vi "FCI Arrow Points.vi"(0 "Max Edge Points":cluster{"X":sgl, "Y":sgl}[](array[cluster]) {"Y" format="%.2f"; "X" format="%.2f"}, 5 "Search Lines":T3[](array[typedef]) {"Edge Info"."Distance (Real-World)" format="%.2f"; "Edge Info"."Location (Real-World)"."Y" format="%.2g"; "Edge Info"."Location (Real-World)"."X" format="%.2f"; "Edge Info"."Noise" format="%.2f"; "Edge Info"."Location (Pixel)"."Y" format="%.2g"; "Edge Info"."Location (Pixel)"."X" format="%.2f"; "Edge Info"."Strength" format="%.2f"; "Edge Info"."Distance (Pixel)" format="%.2f"}, 7 "Edge Last Points":cluster{"X":sgl, "Y":sgl}[](array[cluster]), 9 "Edge First Points":cluster{"X":sgl, "Y":sgl}[](array[cluster]), 11 "error constant":errorcluster) -> (6 "First Arrow Line Coord":T1, 8 "Second Arrow Line Coord":T2, 13 "Max first Arrow Line Coord out":T1, 14 "Max Last Arrow Line Coord out":T1, 15 "error IO":errorcluster)   [LabVIEW 2019, in "Algorithm.lvclass"]
uses:
  FrameworkOverrides/Algorithm.lvclass
  <vilib>/vision/Measure.llb/Edge New.ctl
  <vilib>/vision/Measure.llb/Search Line.ctl
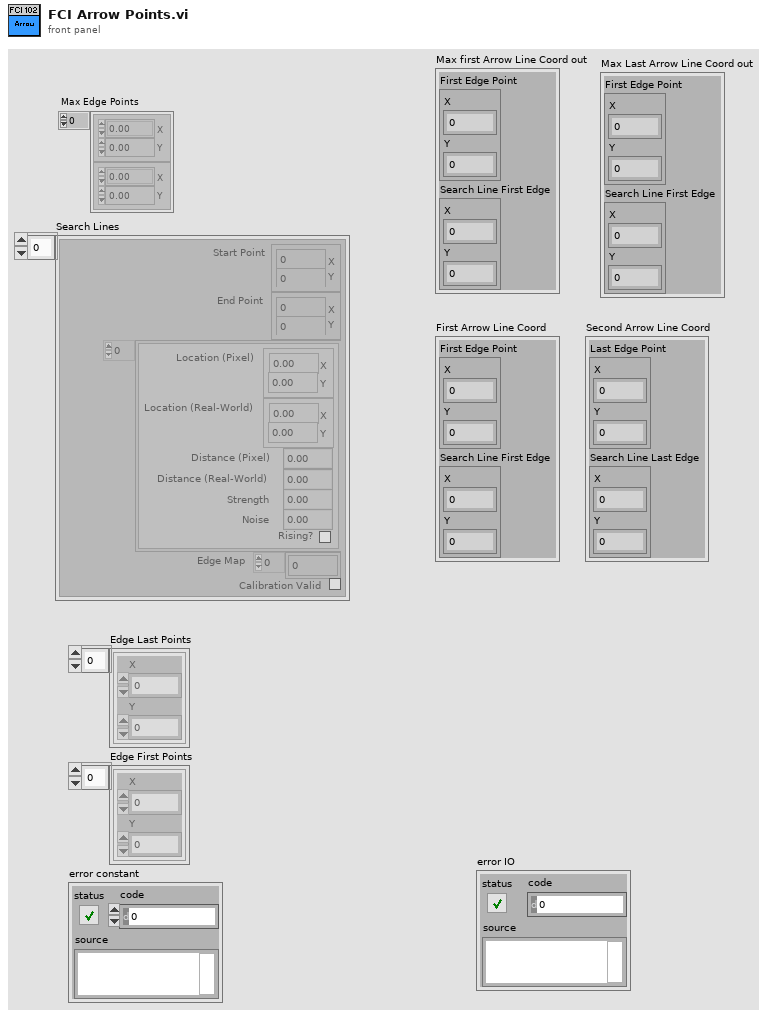
[diagram p1: front panel]
types:
  T1 = cluster{"First Edge Point":cluster{"X":sgl, "Y":sgl}, "Search Line First Edge":cluster{"X":sgl, "Y":sgl}}
  T2 = cluster{"Last Edge Point":cluster{"X":sgl, "Y":sgl}, "Search Line Last Edge":cluster{"X":sgl, "Y":sgl}}
  T3 = typedef "Search Line.ctl" = cluster{"Start Point":cluster{"X":sgl, "Y":sgl}, "End Point":cluster{"X":sgl, "Y":sgl}, "Edge Info":T4[], "Edge Map":dbl[], "Calibration Valid":bool}
  T4 = typedef "Edge New.ctl" = cluster{"Location (Pixel)":cluster{"X":sgl, "Y":sgl}, "Location (Real-World)":cluster{"X":sgl, "Y":sgl}, "Distance (Pixel)":dbl, "Distance (Real-World)":dbl, "Strength":dbl, "Noise":dbl, "Rising?":bool}
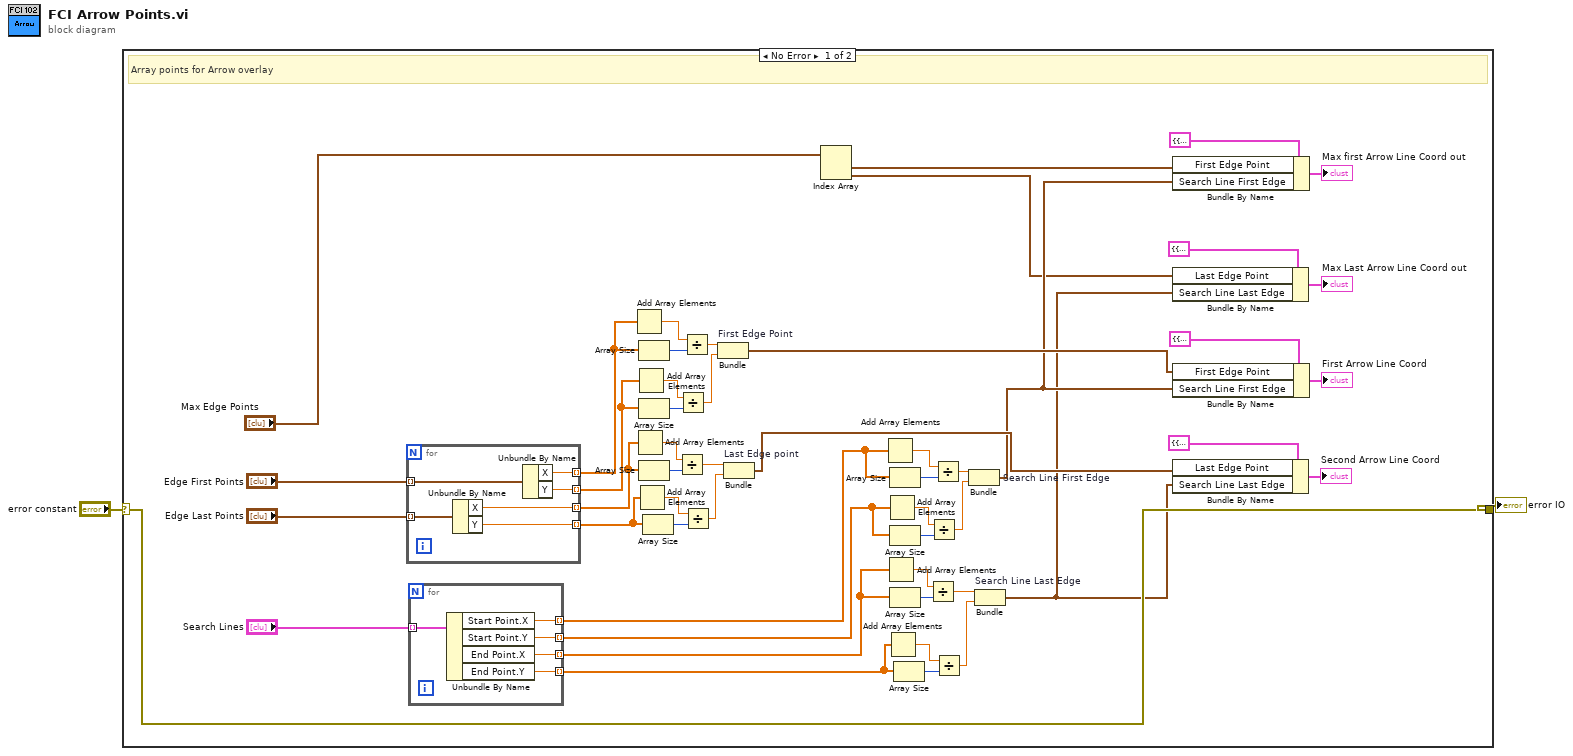
[diagram p0: block diagram]
diagram:
  n1 = case shown="No Error" "error constant" {
    selector: "error constant" -> [w18 w65]
    tunnel: [w18 w65] -> w1
    frame No Error {
      # "Array points for Arrow overlay"
      n2 = for {
        tunnel: "Edge Last Points" -> [w63] mode=indexing
        tunnel: "Edge First Points" -> [w64] mode=indexing
        tunnel: [w62] -> w37 mode=indexing
        tunnel: [w61] -> w41 mode=indexing
        tunnel: [w60] -> w46 mode=indexing
        tunnel: [w59] -> w50 mode=indexing
        n3 = Unbundle By Name(w63) -> ("X"=w60:sgl, "Y"=w59:sgl)
        n4 = Unbundle By Name(w64) -> ("X"=w62:sgl, "Y"=w61:sgl)
      }
      n5 = for {
        tunnel: "Search Lines" -> [w58] mode=indexing
        tunnel: [w57] -> w22 mode=indexing
        tunnel: [w56] -> w21 mode=indexing
        tunnel: [w55] -> w20 mode=indexing
        tunnel: [w54] -> w19 mode=indexing
        n6 = Unbundle By Name(w58) -> ("Start Point.X"=w57:sgl, "Start Point.Y"=w56:sgl, "End Point.X"=w55:sgl, "End Point.Y"=w54:sgl)
      }
      n7 = Add Array Elements(numeric array=w37) -> (sum=w36:sgl)
      n8 = Add Array Elements(numeric array=w46) -> (sum=w44:sgl)
      n9 = Add Array Elements(numeric array=w41) -> (sum=w40:sgl)
      n10 = Add Array Elements(numeric array=w50) -> (sum=w48:sgl)
      n11 = Array Size(array=w37) -> (size(s)=w38:i32)
      n12 = Array Size(array=w41) -> (size(s)=w42:i32)
      n13 = Array Size(array=w46) -> (size(s)=w45:i32)
      n14 = Array Size(array=w50) -> (size(s)=w49:i32)
      n15 = Divide(x=w44, y=w45) -> (x/y=w43:sgl)
      n16 = Divide(x=w40, y=w42) -> (x/y=w39:sgl)
      n17 = Divide(x=w36, y=w38) -> (x/y=w35:sgl)
      n18 = Divide(x=w48, y=w49) -> (x/y=w47:sgl)
      n19 = Bundle "First Edge Point"(w35, w39) -> (w16:cluster{sgl, sgl})  [unwired: 1 in]
      n20 = Bundle "Last Edge point"(w43, w47) -> (w14:cluster{sgl, sgl})  [unwired: 1 in]
      n21 = Index Array(array="Max Edge Points") -> (element #1=w5:cluster{"X":sgl, "Y":sgl}, element #2=w4:cluster{"X":sgl, "Y":sgl})  [unwired: 2 in]
      n22 = Add Array Elements(numeric array=w22) -> (sum=w33:sgl)
      n23 = Add Array Elements(numeric array=w20) -> (sum=w27:sgl)
      n24 = Add Array Elements(numeric array=w21) -> (sum=w30:sgl)
      n25 = Add Array Elements(numeric array=w19) -> (sum=w24:sgl)
      n26 = Array Size(array=w22) -> (size(s)=w32:i32)
      n27 = Array Size(array=w21) -> (size(s)=w29:i32)
      n28 = Array Size(array=w20) -> (size(s)=w26:i32)
      n29 = Array Size(array=w19) -> (size(s)=w23:i32)
      n30 = Divide(x=w27, y=w26) -> (x/y=w28:sgl)
      n31 = Divide(x=w30, y=w29) -> (x/y=w31:sgl)
      n32 = Divide(x=w33, y=w32) -> (x/y=w34:sgl)
      n33 = Divide(x=w24, y=w23) -> (x/y=w25:sgl)
      n34 = Bundle "Search Line First Edge"(w34, w31) -> (w8:cluster{sgl, sgl})  [unwired: 1 in]
      n35 = Bundle "Search Line Last Edge"(w28, w25) -> (w7:cluster{sgl, sgl})  [unwired: 1 in]
      n36 = Bundle By Name(cluster=T1 {"First Edge Point"={"X"=0.0, "Y"=0.0}, "Search Line First Edge"={"X"=0.0, "Y"=0.0}} ("Line Coordinates"), "First Edge Point"=w5, "Search Line First Edge"=w8) -> (→"Max first Arrow Line Coord out":T1)
      n37 = Bundle By Name(cluster=T2 {"Last Edge Point"={"X"=0.0, "Y"=0.0}, "Search Line Last Edge"={"X"=0.0, "Y"=0.0}} ("Line Coordinates"), "Last Edge Point"=w4, "Search Line Last Edge"=w7) -> (→"Max Last Arrow Line Coord out":T2)
      n38 = Bundle By Name(cluster=T1 {"First Edge Point"={"X"=0.0, "Y"=0.0}, "Search Line First Edge"={"X"=0.0, "Y"=0.0}} ("Line Coordinates"), "First Edge Point"=w16, "Search Line First Edge"=w8) -> (→"First Arrow Line Coord":T1)
      n39 = Bundle By Name(cluster=T2 {"Last Edge Point"={"X"=0.0, "Y"=0.0}, "Search Line Last Edge"={"X"=0.0, "Y"=0.0}} ("Line Coordinates"), "Last Edge Point"=w14, "Search Line Last Edge"=w7) -> (→"Second Arrow Line Coord":T2)
    }
    frame Error {
    }
  }
  "error IO" <- w1
